vi "MotionMagicDrive.vi"(1 "Enable Vision Y":bool, 4 "X offset":dbl format="%#_13g", 5 "High gear?":bool, 6 "Y offset":dbl format="%#_13g", 7 "Enable Vision X":bool, 8 "error in (no error)":errorcluster, 9 "Y Axis":dbl, 10 "X Axis":dbl, 11 "Pod Drive in":refnum<class "Pod Drive.lvclass">) -> (0 "error out":errorcluster, 3 "Pod Drive out":refnum<class "Pod Drive.lvclass">)   [LabVIEW 2019, in "DriveOld.lvlib" / "Pod Drive.lvclass"]
doc: "This VI alows you to swich between motion magic GoTo and Closed Loop"
uses:
  Pod Drive.lvclass
  Controls/Mode.ctl
  Drive.lvclass
panel:
  in  "Xmultiplyer":dbl=70.0 format="%#_13g"
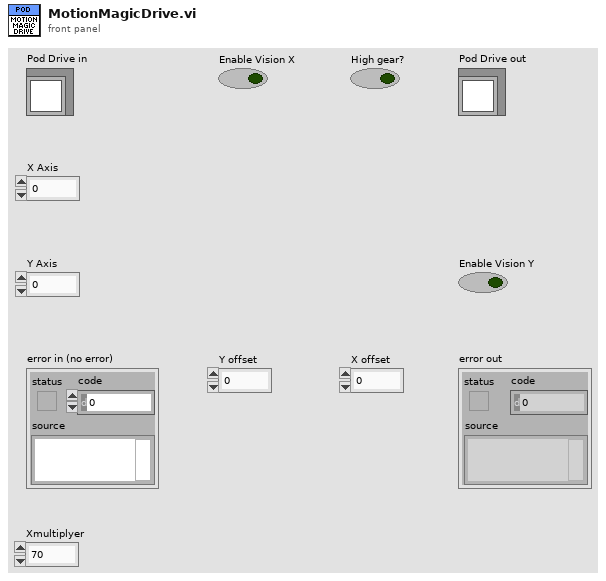
[diagram p1: front panel]
types:
  T1 = typedef "DriveOld.lvlib/Pod Drive.lvclass/Mode.ctl" = enum16{"ClosedLoop", "MotionMagic"}
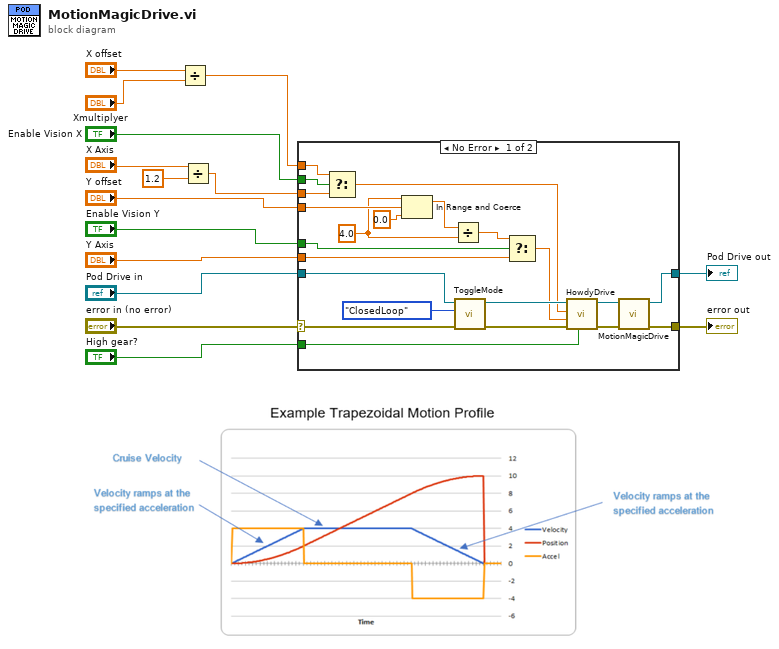
[diagram p0: block diagram]
diagram:
  n1 = Divide(x="X offset", y="Xmultiplyer") -> (x/y=w7:dbl)
  n2 = Divide(x="X Axis", y=1.2) -> (x/y=w1:dbl)
  n3 = case shown="No Error" "error in (no error)" {
    selector: "error in (no error)" -> [w33 w38]
    tunnel: [w37 w38] -> w15
    tunnel: [w36 w39] -> w14
    tunnel: "Pod Drive in" -> [w32 w39]
    tunnel: "Enable Vision X" -> [w26 _]
    tunnel: w1 -> [w30 _]
    tunnel: w7 -> [w25 _]
    tunnel: "Y Axis" -> [w22 _]
    tunnel: "High gear?" -> [w29 _]
    tunnel: "Enable Vision Y" -> [w21 _]
    tunnel: "Y offset" -> [w19 _]
    frame No Error {
      w17 = 4.0 ("upper limit")
      n4 = Select(t=w25, s=w26, f=w30) -> (s? t:f=w24:dbl)
      n5 = In Range and Coerce(upper limit=w17, x=w19, lower limit=0.0) -> (coerced(x)=w18:dbl)  [unwired: 1 out]
      n6 = Divide(x=w18, y=w17) -> (x/y=w16:dbl)
      n7 = call-dynamic "ToggleMode.vi"("error in (no error)"=w33, "Mode"=Mode."ClosedLoop" ("ClosedLoopOrMotionMagic"), "Pod Drive in"=w32) -> ("error out"=w28:errorcluster, "Pod Drive out"=w31:refnum<class "Pod Drive.lvclass">)  [unwired: 7 in]
      n8 = Select(t=w16, s=w21, f=w22) -> (s? t:f=w23:dbl)
      n9 = call-dynamic "HowdyDrive.vi"("HighGear?"=w29, "error in (no error)"=w28, "Y"=w23, "X"=w24, "Pod Drive in"=w31) -> ("error out"=w34:errorcluster, "Pod Drive out"=w35:refnum<class "Pod Drive.lvclass">)  [unwired: 5 in]
      n10 = call-parent "MotionMagicDrive.vi"("error in (no error)"=w34, "Drive in"=w35) -> ("error out"=w37:errorcluster, "Drive out"=w36:refnum<class "Pod Drive.lvclass">)  [unwired: 8 in]
    }
    frame Error {
    }
  }
  "error out" <- w15
  "Pod Drive out" <- w14
